vi "Max Read Array.vi"(8 "error in":errorcluster, 11 "Max Humidity Limit in":refnum<class "Humidity Limit.lvclass">) -> (0 "error out":errorcluster, 1 "Changed or First Call?":bool, 2 "Humidity Max SP":dbl[](array[numeric]), 3 "Max Humidity Limit out":refnum<class "Humidity Limit.lvclass">)   [LabVIEW 2023, in "Humidity Limit.lvclass"]
uses:
  Humidity Limit.lvclass
  Humidity Limit.lvclass/Humidity Limit.ctl
  Parents/Limit/Limit.lvclass
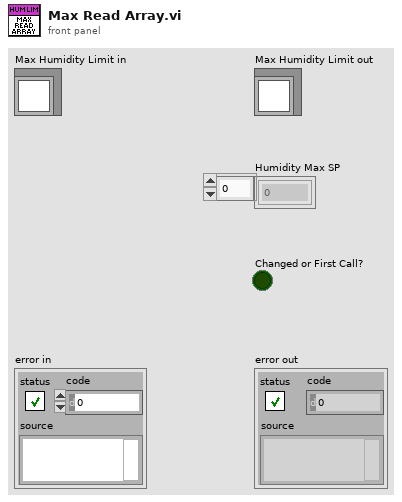
[diagram p1: front panel]
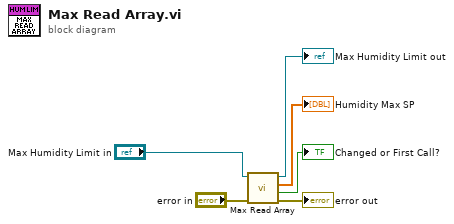
[diagram p0: block diagram]
diagram:
  n1 = call-parent "Max Read Array.vi"("error in"="error in", "Max Limit in"="Max Humidity Limit in") -> ("error out"=→"error out":errorcluster, "Changed or First Call?"=→"Changed or First Call?":bool, "Current Max SP"=→"Humidity Max SP":dbl[], "Max Limit out"=→"Max Humidity Limit out":refnum<class "Humidity Limit.lvclass">)  [unwired: 6 in]
